vi "Sample_SimpleStructRead.vi"() -> ()   [LabVIEW 2022 SP3]
uses:
  TypeDefs/EL92xxOCPInputs.ctl
panel:
  out "OCP Inputs":T1
  out "RData":variant
  out "Read status?":bool
  in  "String":string
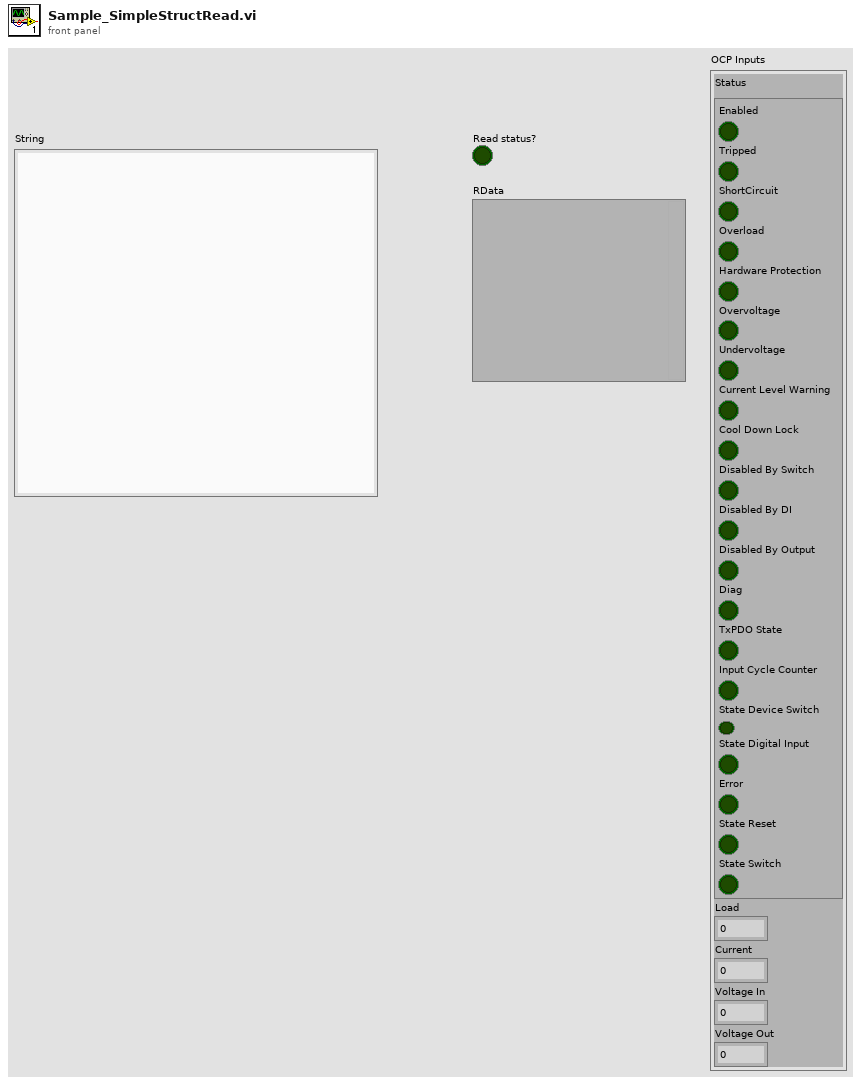
[diagram p1: front panel]
types:
  T1 = typedef "EL92xxOCPInputs.ctl" = cluster{"Status":cluster{"Enabled":bool, "Tripped":bool, "ShortCircuit":bool, "Overload":bool, "Hardware Protection":bool, "Overvoltage":bool, "Undervoltage":bool, "Current Level Warning":bool, "Cool Down Lock":bool, "Disabled By Switch":bool, "Disabled By DI":bool, "Disabled By Output":bool, "Diag":bool, "TxPDO State":bool, "Input Cycle Counter":bool, "State Device Switch":bool, "State Digital Input":bool, "Error":bool, "State Reset":bool, "State Switch":bool}, "Load":dbl, "Current":dbl, "Voltage In":dbl, "Voltage Out":dbl}
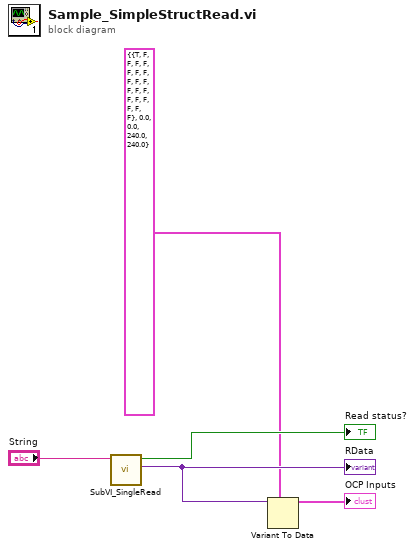
[diagram p0: block diagram]
diagram:
  n1 = call "SubVI_SingleRead.vi"("String"="String") -> ("RData"=w3:variant, "Read status?"=→"Read status?":bool)  [unwired: 7 in, 1 out]
  "RData" <- w3
  n2 = Variant To Data(type=T1 {"Status"={"Enabled"=TRUE, "Tripped"=FALSE, "ShortCircuit"=FALSE, "Overload"=FALSE, "Hardware Protection"=FALSE, "Overvoltage"=FALSE, "Undervoltage"=FALSE, "Current Level Warning"=FALSE, "Cool Down Lock"=FALSE, "Disabled By Switch"=FALSE, "Disabled By DI"=FALSE, "Disabled By Output"=FALSE, "Diag"=FALSE, "TxPDO State"=FALSE, "Input Cycle Counter"=FALSE, "State Device Switch"=FALSE, "State Digital Input"=FALSE, "Error"=FALSE, "State Reset"=FALSE, "State Switch"=FALSE}, "Load"=0.0, "Current"=0.0, "Voltage In"=240.0, "Voltage Out"=240.0} ("OCP Inputs"), Variant=w3) -> (data=→"OCP Inputs":T1)  [unwired: 1 in, 1 out]
